vi "Read HP Freq.vi"() -> (0 "Frequency (GHz)":dbl format="%.3f")   [LabVIEW 2010]
uses:
  MWC Global.vi
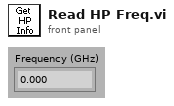
[diagram p1: front panel]
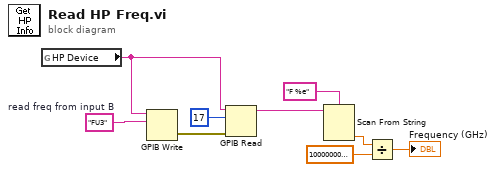
[diagram p0: block diagram]
diagram:
  w9 = "FU3"  # read freq from input B
  n1 = global read "MWC Global.vi" "HP Device"() -> (w6:string)
  n2 = GPIB Write(0:w6, 1:w9) -> (6:w8:errorcluster)  [unwired: 3 in, 1 out]
  n3 = GPIB Read(0:w6, 1:17 ("byte count"), 3:w8) -> (5:w5:string)  [unwired: 2 in, 2 out]
  n4 = Scan From String(format string="F %e", input string=w5) -> (output 1=w3:dbl)  [unwired: 3 in, 3 out]
  n5 = Divide(x=w3, y=1000000000.0) -> (x/y=→"Frequency (GHz)":dbl)
